vi "UART_Burst&Capture.vi"(6 "timeout (s)":dbl=10.0, 7 "site list":string, 8 "error in (no error)":errorcluster, 9 "Reply Bytes":i32, 10 "start label":string="uart", 11 "IVI Refnum in":refnum<k15>) -> (0 "error out":errorcluster, 1 "pass":bool[](array[boolean]), 2 "Data Out":u8[](array[numeric]), 3 "IVI Refnum out":refnum<k15>)   [LabVIEW 2024, in "UART.lvlib"]
doc: "Burst the pattern and captures data from uart_capture waveform"
uses:
  UART.lvlib
  <instrlib>/niDigital/niDigital.llb/niDigital Burst Pattern (Pass Fail).vi
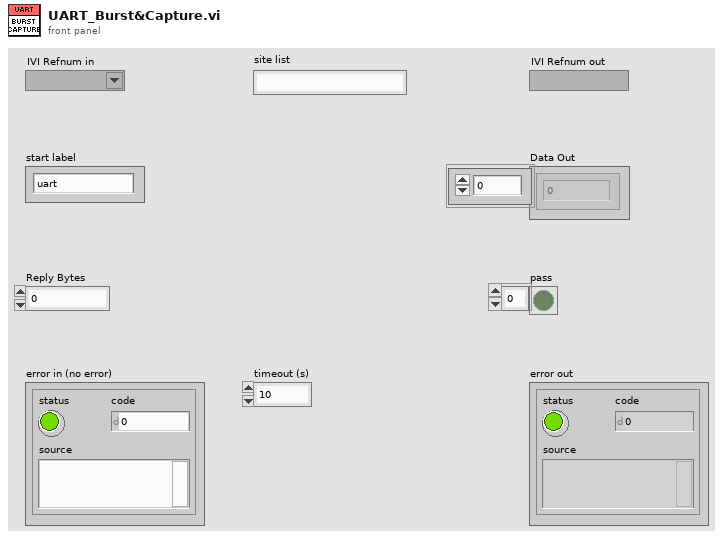
[diagram p1: front panel]
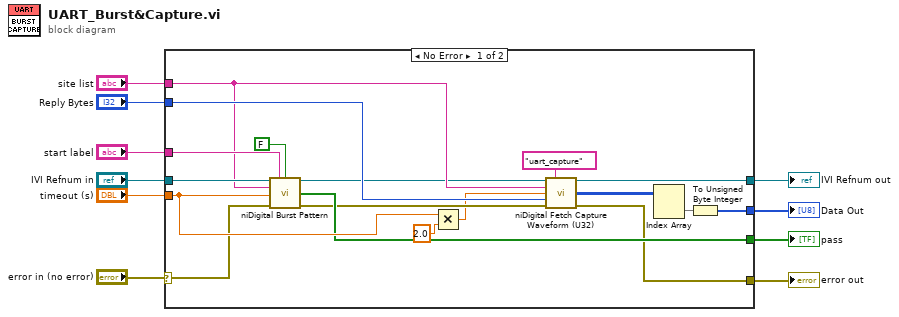
[diagram p0: block diagram]
diagram:
  n1 = case shown="No Error" "error in (no error)" {
    selector: "error in (no error)" -> [w21 w30]
    tunnel: [w28 w29] -> w10
    tunnel: "IVI Refnum in" -> [w27 w29]
    tunnel: "start label" -> [w26 _]
    tunnel: "Reply Bytes" -> [w25 _]
    tunnel: [w24 _] -> w6
    tunnel: "site list" -> [w23 _]
    tunnel: [w20 _] -> w4
    tunnel: "timeout (s)" -> [w22 _]
    tunnel: [w19 w30] -> w2
    frame No Error {
      n2 = call-poly <instrlib>:"niDigital Burst Pattern.vi"("instrument handle"=w27, "start label"=w26, "select digital function? (T)"=FALSE, "site list"=w23, "timeout (s)"=w22, "error in"=w21) -> ("instrument handle out"=w18:refnum<k15>, "pass"=w20:bool[], "error out"=w16:errorcluster)  [unwired: 7 in]
      n3 = Multiply(x=w22, y=2.0) -> (x*y=w14:dbl)
      n4 = call <instrlib>:"niDigital Fetch Capture Waveform (U32).vi"("instrument handle"=w18, "waveform name"="uart_capture", "site list"=w23, "timeout (s)"=w14, "samples to read"=w25, "error in"=w16) -> ("instrument handle out"=w28:refnum<k15>, "data"=w12:u32[][], "error out"=w19:errorcluster)  [unwired: 7 in]
      n5 = Index Array(array=w12) -> (element=w11:u32[])  [unwired: 2 in]
      n6 = To Unsigned Byte Integer(number=w11) -> (unsigned 8bit integer=w24:u8[])
    }
    frame Error {
    }
  }
  "IVI Refnum out" <- w10
  "error out" <- w2
  "Data Out" <- w6
  "pass" <- w4
